vi "Tutorial 09.vi"() -> ()   [LabVIEW 2014]
panel:
  out "Loop Number":i32
  out "Random Number":dbl
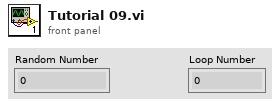
[diagram p1: front panel]
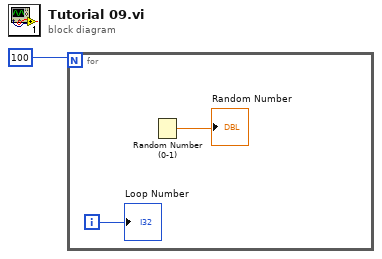
[diagram p0: block diagram]
diagram:
  n1 = for {
    N: 100 -> [_]
    i -> [w2]
    n2 = Random Number (0-1)() -> (number: 0 to 1=→"Random Number":dbl)
    "Loop Number" <- w2
  }
